vi "UMLEditor GetCallersWorkingDirectory.vi"(8 "error in (no error)":errorcluster, 11 "Get the top VI's Info(False)":bool) -> (0 "error out":errorcluster, 2 "VI name":string, 3 "VI directory":path)   [LabVIEW 2016]
doc: "This VI returns the working director of this VIs caller.\nIt works even when running in an llb or in a exe-file.\nIt also return the VI name of the caller."
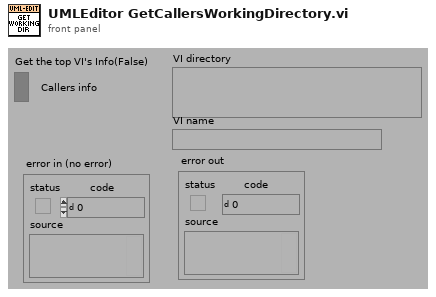
[diagram p1: front panel]
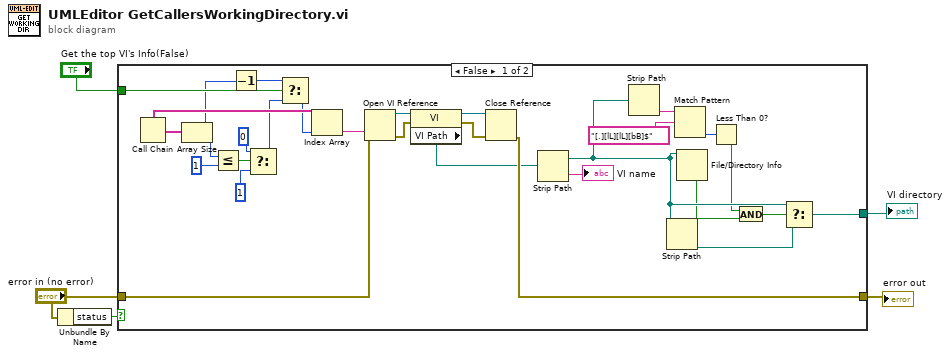
[diagram p0: block diagram]
diagram:
  n1 = Unbundle By Name("error in (no error)") -> ("status"=w4:bool)
  n2 = case shown="False" w4 {
    tunnel: "error in (no error)" -> [w21 w34]
    tunnel: [w20 w34] -> w3
    tunnel: "Get the top VI's Info(False)" -> [w18 _]
    tunnel: [w13 _] -> w1
    frame False {
      n3 = Call Chain() -> (call chain=w22:string[])
      n4 = Array Size(array=w22) -> (size(s)=w15:i32)
      n5 = Less Or Equal?(x=w15, y=1) -> (x <= y?=w23:bool)
      n6 = Decrement(x=w15) -> (x-1=w14:i32)
      n7 = Select(t=0, s=w23, f=1) -> (s? t:f=w16:i32)
      n8 = Select(t=w14, s=w18, f=w16) -> (s? t:f=w17:i32)
      n9 = Index Array(array=w22, index=w17) -> (element=w26:string)
      n10 = Open VI Reference(vi path=w26, error in (no error)=w21) -> (vi reference=w27:refnum<vi>, error out=w29:errorcluster)  [unwired: 4 out]
      n11 = property class="VI"(reference=w27, error in=w29) -> (reference out=w28:refnum<vi>, error out=w30:errorcluster, "VI Path"=w19:path)
      n12 = Close Reference(reference=w28, error in (no error)=w30) -> (error out=w20:errorcluster)
      n13 = Strip Path(path=w19) -> (stripped path=w12:path, name=→"VI name":string)
      n14 = Strip Path(path=w12) -> (name=w11:string)  [unwired: 1 out]
      n15 = Strip Path(path=w12) -> (stripped path=w33:path)  [unwired: 1 out]
      n16 = Match Pattern(string=w11, regular expression="[.][lL][lL][bB]$") -> (offset past match=w9:i32)  [unwired: 4 out]
      n17 = File/Directory Info(path=w12) -> (directory=w7:bool)  [unwired: 1 in, 6 out]
      n18 = Less Than 0?(x=w9) -> (x < 0?=w6:bool)
      n19 = And(x=w6, y=w7) -> (x .and. y?=w8:bool)
      n20 = Select(t=w12, s=w8, f=w33) -> (s? t:f=w13:path)
    }
    frame True {
    }
  }
  "error out" <- w3
  "VI directory" <- w1
